vi "Update HTML File.vi"(10 "Data In":T1, 11 "Path":path) -> (3 "URL out":string)   [LabVIEW 2016, in "Line Chart.xctl"]
uses:
  Line Chart.xctl
  Data Line Chart.ctl
panel:
  out "error out":errorcluster
  # "D:\\Ultratech\\Bitbucket\\Log Plotter\\xcontrol\\js"
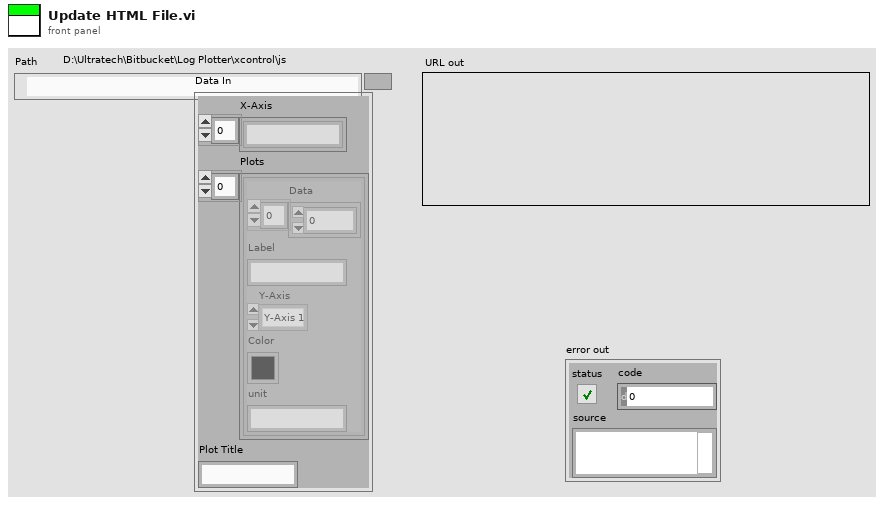
[diagram p1: front panel]
types:
  T1 = typedef "Line Chart.xctl/Data Line Chart.ctl" = cluster{"X-Axis":string[], "Plots":cluster{"Data":dbl[], "Label":string, "Y-Axis":enum16{"Y-Axis 1", "Y-Axis 2", "Y-Axis 3", "Y-Axis 4", "Y-Axis 5", "Y-Axis 6", "Y-Axis 7", "Y-Axis 8", "Y-Axis 9", "Y-Axis 10"}, "Color":u32, "unit":string}[], "Plot Title":string}
  T2 = enum16{"open", "replace", "create", "open or create", "replace or create", "replace or create with confirmation"}
  T3 = cluster{"Data":dbl[], "Label":string, "Y-Axis":enum16{"Y-Axis 1", "Y-Axis 2", "Y-Axis 3", "Y-Axis 4", "Y-Axis 5", "Y-Axis 6", "Y-Axis 7", "Y-Axis 8", "Y-Axis 9", "Y-Axis 10"}, "Color":u32, "unit":string}[]
  T4 = enum16{"Y-Axis 1", "Y-Axis 2", "Y-Axis 3", "Y-Axis 4", "Y-Axis 5", "Y-Axis 6", "Y-Axis 7", "Y-Axis 8", "Y-Axis 9", "Y-Axis 10"}
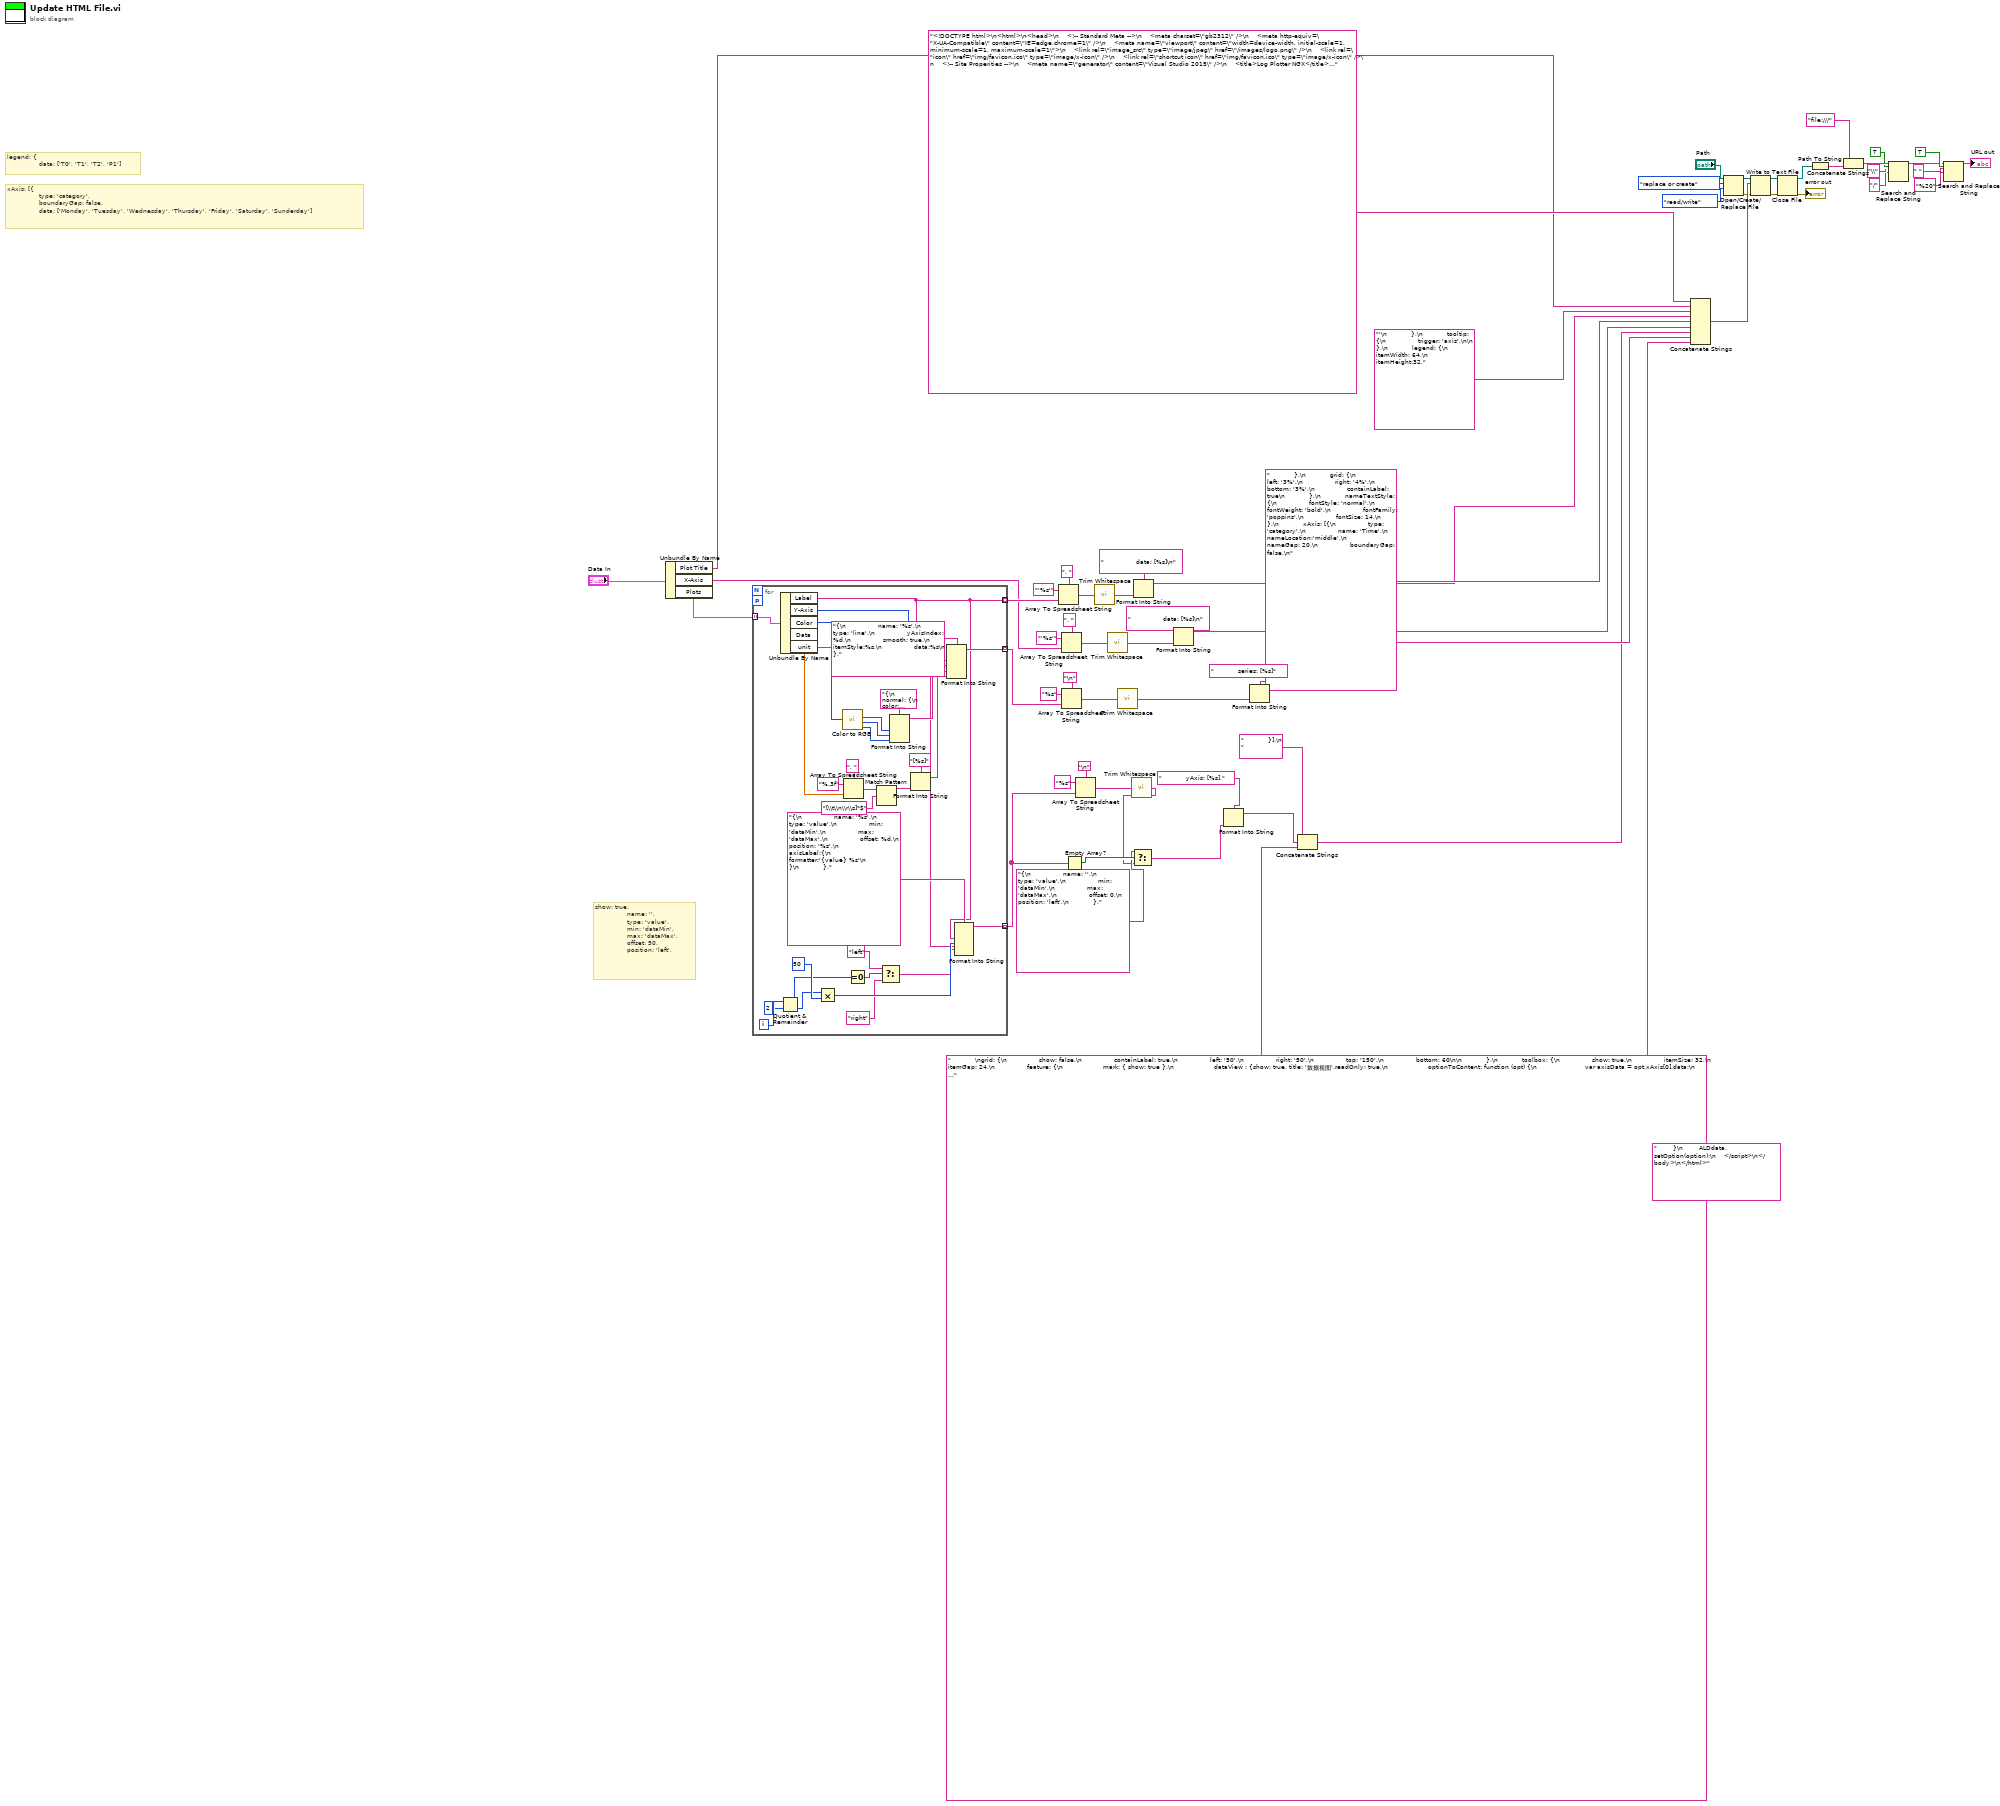
[diagram p0: block diagram]
diagram:
  # "show: true,\n                name: '',\n                type: 'value',\n                min: 'dataMin',\n                max: 'dataMax',\n                offset: 50,\n                position: 'left',"
  # "xAxis: [{\n                type: 'category',\n                boundaryGap: false,\n                data: ['Monday', 'Tuesday', 'Wednesday', 'Thursday', 'Friday', 'Saturday', 'Sunderday']"
  # "legend: {\n                data: ['T0', 'T1', 'T2', 'P1']"
  n1 = Unbundle By Name("Data In") -> ("Plot Title"=w15:string, "X-Axis"=w56:string[], "Plots"=w62:T3)
  n2 = for {
    tunnel: w62 -> [w94] mode=indexing
    tunnel: [w73] -> w61 mode=indexing
    tunnel: [w82] -> w55 mode=indexing
    workers-P: _ -> [_]
    tunnel: [w64] -> w5 mode=indexing
    i -> [w75]
    n3 = Unbundle By Name(w94) -> ("Label"=w73:string, "Y-Axis"=w84:T4, "Color"=w90:u32, "Data"=w93:dbl[], "unit"=w63:string)
    n4 = Quotient & Remainder(x=w75, y=2) -> (x-y*floor(x/y)=w69:i32, floor(x/y)=w70:i32)
    n5 = Multiply(x=w70, y=50) -> (x*y=w71:i32)
    n6 = call <vilib>:"Color to RGB.vi"("Color"=w90) -> ("R"=w88:u8, "G"=w87:u8, "B"=w86:u8)  [unwired: 1 out]
    n7 = Array To Spreadsheet String(delimiter (Tab)=", ", array=w93, 3:"%.3f" ("format string")) -> (spreadsheet string=w79:string)
    n8 = Equal To 0?(x=w69) -> (x = 0?=w68:bool)
    n9 = Match Pattern(string=w79, regular expression="[\\t\\n\\r\\s]*$") -> (before substring=w78:string)  [unwired: 1 in, 3 out]
    n10 = Select(t="left", s=w68, f="right") -> (s? t:f=w65:string)
    n11 = Format Into String(format string="{\n                    normal: {\n                        color: 'rgba(%d, %d,%d,10)',\n                            }\n                }", w88, w87, w86) -> (resulting string=w83:string)  [unwired: 2 in, 1 out]
    n12 = Format Into String(format string="[%s]", w78) -> (resulting string=w80:string)  [unwired: 2 in, 1 out]
    n13 = Format Into String(format string="{\n                name: '%s',\n                type: 'line',\n                yAxisIndex: %d,\n                smooth: true,\n                itemStyle:%s,\n                data:%s\n            },", w73, w84, w83, w80) -> (resulting string=w82:string)  [unwired: 2 in, 1 out]
    n14 = Format Into String(format string="{\n                name: '%s',\n                type: 'value',\n                min: 'dataMin',\n                max: 'dataMax',\n                offset: %d,\n                position: '%s',\n                axisLabel:{\n                    formatter:'{value} %s'\n                }\n            },", w73, w71, w65, w63) -> (resulting string=w64:string)  [unwired: 2 in, 1 out]
  }
  n15 = Array To Spreadsheet String(delimiter (Tab)=", ", array=w61, 3:"'%s'" ("format string")) -> (spreadsheet string=w49:string)
  n16 = Array To Spreadsheet String(delimiter (Tab)=", ", array=w56, 3:"'%s'" ("format string")) -> (spreadsheet string=w46:string)
  n17 = Array To Spreadsheet String(delimiter (Tab)="\n", array=w55, 3:"%s" ("format string")) -> (spreadsheet string=w43:string)
  n18 = Empty Array?(array=w5) -> (empty?=w4:bool)
  n19 = Array To Spreadsheet String(delimiter (Tab)="\n", array=w5, 3:"%s" ("format string")) -> (spreadsheet string=w13:string)
  n20 = call <vilib>:"Trim Whitespace.vi"("string"=w49) -> ("trimmed string"=w41:string)  [unwired: 1 in]
  n21 = call <vilib>:"Trim Whitespace.vi"("string"=w46) -> ("trimmed string"=w40:string)  [unwired: 1 in]
  n22 = call <vilib>:"Trim Whitespace.vi"("string"=w43) -> ("trimmed string"=w39:string)  [unwired: 1 in]
  n23 = call <vilib>:"Trim Whitespace.vi"("string"=w13) -> ("trimmed string"=w1:string)  [unwired: 1 in]
  n24 = Select(t="{\n                name: '',\n                type: 'value',\n                min: 'dataMin',\n                max: 'dataMax',\n                offset: 0,\n                position: 'left',\n            },", s=w4, f=w1) -> (s? t:f=w2:string)
  n25 = Format Into String(format string="                data: [%s]\n", w41) -> (resulting string=w48:string)  [unwired: 2 in, 1 out]
  n26 = Format Into String(format string="                data: [%s]\n", w40) -> (resulting string=w45:string)  [unwired: 2 in, 1 out]
  n27 = Format Into String(format string="            yAxis: [%s],", w2) -> (resulting string=w9:string)  [unwired: 2 in, 1 out]
  n28 = Format Into String(format string="            series: [%s]", w39) -> (resulting string=w42:string)  [unwired: 2 in, 1 out]
  n29 = Concatenate Strings("            }],\n            ", w9, "            \ngrid: {\n                show: false,\n                containLabel: true,\n                left: '50',\n                right: '50',\n                top: '150',\n                bottom: 60\n\n            },\n            toolbox: {\n                show: true,\n                itemSize: 32,\n                itemGap: 24,\n                feature: {\n                    mark: { show: true },\n                    dataView : {show: true, title: '数据视图',readOnly: true,\n                    optionToContent: function (opt) {\n                        var axisData = opt.xAxis[0].data;\n                        var series = opt.series;\n                        var tdHeads = '<td  style=\"padding:12px 28px\">时间</td>';\n                        series.forEach(function (item) {\n                            tdHeads += '<td style=\"padding: 12px 28px\">'+item.name+'</td>';\n                        });\n                        var table = '<div style=\"height:100%;overflow:scroll;\"><table border=\"1\" style=\"margin:12 28;border-collapse:collapse;font-size:24px;text-align:center\"><tbody><tr>'+tdHeads+'</tr>';\n                        var tdBodys = '';\n                        for (var i = 0, l = axisData.length; i < l; i++) {\n                            for (var j = 0; j < series.length; j++) {\n                                if(typeof(series[j].data[i]) == 'object'){\n                                    tdBodys += '<td>'+series[j].data[i].value+'</td>';\n                                }else{\n                                    tdBodys += '<td>'+ series[j].data[i]+'</td>';\n                                }\n                            }\n                            table += '<tr><td style=\"padding: 12px 28px\">'+axisData[i]+'</td>'+ tdBodys +'</tr>';\n                            tdBodys = '';\n                        }\n                            table += '</tbody></table></div>';\n                            return table;\n                    }\n            },\n                    magicType: { show: true, title:{line:'折线图',bar:'柱状图',},type: ['line', 'bar'] },\n                    restore: { show: true, title: '刷新' },\n                    saveAsImage: { show: true, title: '保存图片',backgroundColor: '#fff' }\n                }\n            },\n            color: [\"#345995\", \"#03CEA4\", \"#FB4D3D\"],\n            dataZoom:[\n                    {\n                        show: true,\n                        type: 'slider',\n                        realtime: true,\n                        start: 0,\n                        end: 100,\n                        height: 50,\n                        handleSize : 50,\n                        bottom: 10,\n                  \n                    },\n                    {\n                        show: true,\n                        type: 'inside',\n                        realtime: true,\n                        start: 0,\n                        end: 100,\n                    },\n            ],\n") -> (w7:string)
  n30 = Concatenate Strings("<!DOCTYPE html>\n<html>\n<head>\n    <!-- Standard Meta -->\n    <meta charset=\"gb2312\" />\n    <meta http-equiv=\"X-UA-Compatible\" content=\"IE=edge,chrome=1\" />\n    <meta name=\"viewport\" content=\"width=device-width, initial-scale=1, minimum-scale=1, maximum-scale=1\">\n    <link rel=\"image_src\" type=\"image/jpeg\" href=\"/images/logo.png\" />\n    <link rel=\"icon\" href=\"img/favicon.ico\" type=\"image/x-icon\" />\n    <link rel=\"shortcut icon\" href=\"img/favicon.ico\" type=\"image/x-icon\" />\n    <!-- Site Properities -->\n    <meta name=\"generator\" content=\"Visual Studio 2015\" />\n    <title>Log Plotter NGX</title>\n    <meta name=\"description\" content=\"Chartli Interactive Chart\" />\n    <meta name=\"keywords\" content=\"html5,chart,ui, library, framework, javascript,jquery,graphic,interactive\" />\n    <link href=\"css/semantic.css\" rel=\"stylesheet\" />\n    <link href=\"css/demo.css\" rel=\"stylesheet\" />\n</head>\n<body>\n\n<div id=\"ALD Data\" style=\"width: 100%;height:100%;\"></div>\n\n    <script src=\"js/jquery-2.1.4.min.js\"></script>\n    <script src=\"js/chartli.js\"></script>\n    <script>\n\n        var ALDdata = echarts.init(document.getElementById('ALD Data'));\n        option = {\n            backgroundColor: '#fffff',\n            color: ['#B33F62', '#F9564F', '#0C0A3E'],\n\n            title: {\n                text: '", w15, "'\n            },\n            tooltip: {\n                trigger: 'axis',\n\n            },\n            legend: {\n                itemWidth: 64,\n                itemHeight:32,", w48, "            },\n            grid: {\n                left: '3%',\n                right: '4%',\n                bottom: '3%',\n                containLabel: true\n            },\n            nameTextStyle: {\n                fontStyle: 'normal',\n                fontWeight: 'bold',\n                fontFamily: 'poppins',\n                fontSize: 14,\n            },\n            xAxis: [{\n                type: 'category',\n                name: 'Time',\n                nameLocation:'middle',\n                nameGap: 20,\n                boundaryGap: false,\n", w45, w7, w42, "        }\n        ALDdata.setOption(option);\n    </script>\n</body>\n</html>") -> (w35:string)
  n31 = Open/Create/Replace File(file path (use dialog)="Path", operation (0:open)=T2."replace or create", access (0:read/write)=enum16{"read/write", "read-only", "write-only"}."read/write") -> (refnum out=w36:refnum<file>, error out=w30:errorcluster)  [unwired: 3 in, 1 out]
  n32 = Write to Text File(file (use dialog)=w36, text=w35, error in=w30) -> (refnum out=w33:refnum<file>, error out=w29:errorcluster)  [unwired: 1 in, 1 out]
  n33 = Close File(refnum=w33, error in=w29) -> (path=w31:path, error out=→"error out":errorcluster)
  n34 = Path To String(path=w31) -> (string=w32:string)
  n35 = Concatenate Strings("file:///" ("string"), w32) -> (w27:string)
  n36 = Search and Replace String(replace all?=TRUE ("replace all? (F)"), input string=w27, search string="\\", replace string="/" ("replace string (\"\")")) -> (result string=w20:string)  [unwired: 4 in, 3 out]
  n37 = Search and Replace String(replace all?=TRUE ("replace all? (F)"), input string=w20, search string=" ", replace string="%20" ("replace string (\"\")")) -> (result string=→"URL out":string)  [unwired: 4 in, 3 out]
